vi "DSF.Engine.Pointer.DBL.Read.vi"(8 "error in (no error)":errorcluster, 10 "buffer in":dbl[](array[numeric]), 11 "DBL Pointer in":refnum<class "DSF.Engine.Pointer.DBL.lvclass">) -> (0 "error out":errorcluster, 2 "buffer out":dbl[](array[numeric]), 3 "DBL Pointer out":refnum<class "DSF.Engine.Pointer.DBL.lvclass">)   [LabVIEW 2017, in "DSF.Engine.lvlib" / "DSF.Engine.Pointer.DBL.lvclass"]
uses:
  DSF.Engine.Pointer.DBL.lvclass
  C:/Git/DSF/dsf core/Built/Windows/Dependencies/Memory Manager.lvlibp/1abvi3w/vi.lib/National Instruments/Memory Manager/Classes/Pointer/Memory.Pointer.lvclass
  DSF.Engine.Pointer.DBL.lvclass/DSF.Engine.Pointer.DBL.ctl
  Built/Windows/Dependencies/Memory Manager.lvlibp/1abvi3w/vi.lib/National Instruments/Memory Manager/Classes/Pointer/Memory.Pointer.Read.1D.DBL.vi
  Built/Windows/Dependencies/Memory Manager.lvlibp/1abvi3w/vi.lib/National Instruments/Memory Manager/Classes/Pointer/Memory.Pointer.lvclass
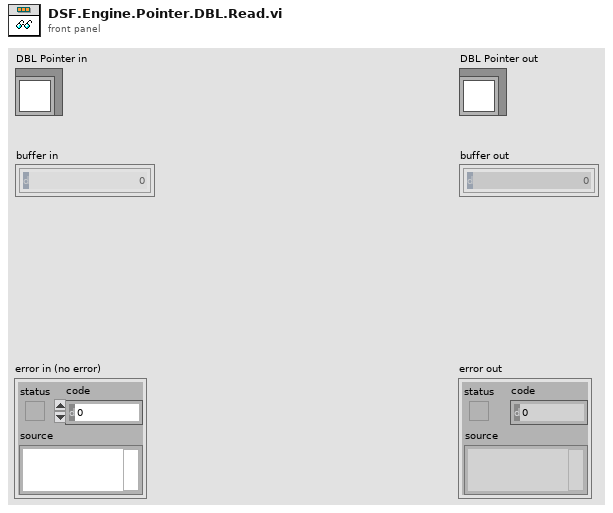
[diagram p1: front panel]
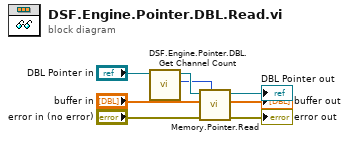
[diagram p0: block diagram]
diagram:
  n1 = call "DSF.Engine.Pointer.DBL.Get Channel Count.vi"("DBL Buffer in"="DBL Pointer in") -> ("channel count"=w3:u64, "DBL Buffer out"=w4:refnum<class "DSF.Engine.Pointer.DBL.lvclass">)  [unwired: 9 in]
  n2 = call-poly "Memory.Pointer.Read.vi"("count (-1: all)"=w3, "error in (no error)"="error in (no error)", "buffer in"="buffer in", "Pointer in"=w4) -> ("error out"=→"error out":errorcluster, "buffer out"=→"buffer out":dbl[], "Pointer out"=→"DBL Pointer out":refnum<class "DSF.Engine.Pointer.DBL.lvclass">)  [unwired: 4 in, 1 out]
